vi "Write.vi"(8 "error in (no error)":errorcluster, 10 "String":string, 11 "Wiresmith CLI Output in":refnum<class "Wiresmith CLI Output.lvclass">) -> (0 "error out":errorcluster, 3 "Wiresmith CLI Output out":refnum<class "Wiresmith CLI Output.lvclass">)   [LabVIEW 2019, in "Wiresmith CLI Output.lvclass"]
uses:
  Wiresmith CLI Output.lvclass
  Wiresmith CLI Output.lvclass/Wiresmith CLI Output.ctl
  <vilib>/Wiresmith Technology/G CLI/CLI Class/CLI.lvclass
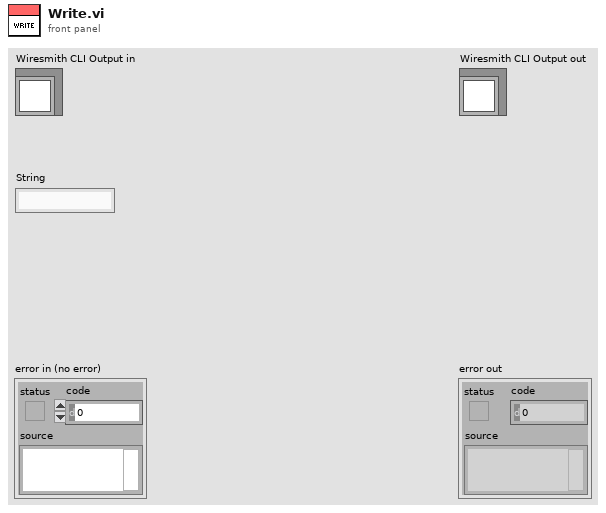
[diagram p1: front panel]
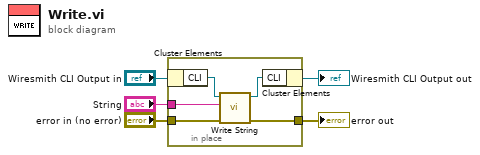
[diagram p0: block diagram]
diagram:
  n1 = in-place {
    in-place-border: "error in (no error)" -> [w8]
    in-place-border: [w7] -> w2
    in-place-border: "String" -> [w6]
    n2 = in-place-cluster #1("Wiresmith CLI Output in") -> ("CLI"=w10:refnum<class "CLI.lvclass">)
    n3 = call <vilib>:"Write String.vi"("error in (no error)"=w8, "Text to Write"=w6, "CLI in"=w10) -> ("error out"=w7:errorcluster, "CLI out"=w9:refnum<class "CLI.lvclass">)  [unwired: 7 in]
    n4 = in-place-cluster #1("CLI"=w9) -> (→"Wiresmith CLI Output out":refnum<class "Wiresmith CLI Output.lvclass">)
  }
  "error out" <- w2
